vi "search hands data.vi"(11 "offset past number":i32) -> (1 "time delay":i32, 3 "hand":T1 {"手臂" scale=0.0..90.0; "转台" scale=0.0..360.0; "拇指" scale=0.0..90.0; "上下移动" scale=0.0..100.0; "食指" scale=0.0..90.0; "中指" scale=0.0..90.0; "无名指" scale=0.0..90.0; "小手指" scale=0.0..90.0; "手腕" scale=0.0..360.0})   [LabVIEW 2016]
uses:
  Controls/robotdata.ctl
  Data Base/StateMachineStates.ctl
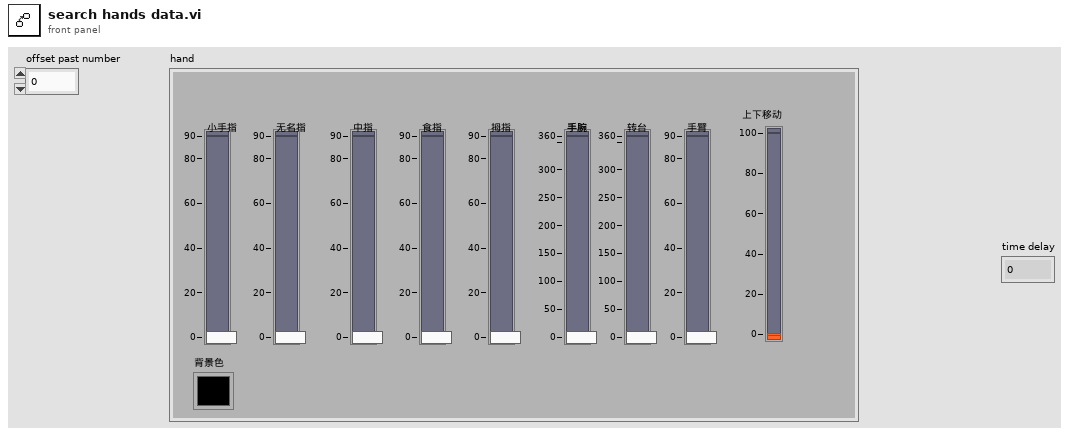
[diagram p1: front panel]
types:
  T1 = typedef "robotdata.ctl" = cluster{"手腕":sgl, "小手指":sgl, "无名指":sgl, "中指":sgl, "食指":sgl, "上下移动":dbl, "背景色":u32, "拇指":sgl, "转台":sgl, "手臂":sgl}
  T2 = typedef "StateMachineStates.ctl" = enum16{"Connection DB", "Creat DB", "Delete Table", "Insert DB", "Inquire Table", "Inquire All DB", "Delete All Data", "Delete Data", "Sort Data", "Inquire Last Data", ""}
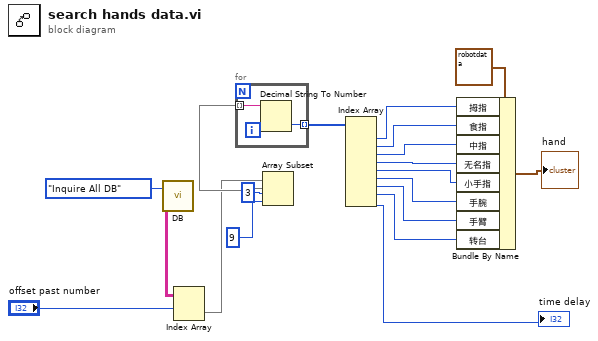
[diagram p0: block diagram]
diagram:
  n1 = call "DB.vi"("Beginning State"=StateMachineStates."Inquire All DB") -> ("Item Data"=w3:string[][])  [unwired: 12 in, 6 out]
  n2 = Index Array(array=w3, index (row)="offset past number") -> (element=w5:string[])  [unwired: 1 in]
  n3 = Array Subset(array=w5, index=3 ("索引"), length=9 ("长度")) -> (w8:string[])
  n4 = for {
    tunnel: w8 -> [w21] mode=indexing
    tunnel: [w20] -> w9 mode=indexing
    n5 = Decimal String To Number(string=w21) -> (number=w20:i32)  [unwired: 2 in, 1 out]
  }
  n6 = Index Array(array=w9) -> (element #1=w11:i32, element #2=w12:i32, element #3=w13:i32, element #4=w14:i32, element #5=w15:i32, element #6=w16:i32, element #7=w17:i32, element #8=w18:i32, element #9=→"time delay":i32)  [unwired: 9 in]
  n7 = Bundle By Name(cluster=T1 {"手腕"=52.38806, "小手指"=0.0, "无名指"=0.0, "中指"=0.0, "食指"=0.0, "上下移动"=-1.8918918918918917, "背景色"=15204350, "拇指"=0.0, "转台"=52.38806, "手臂"=52.38806} ("hand"), "拇指"=w11, "食指"=w12, "中指"=w13, "无名指"=w14, "小手指"=w15, "手腕"=w16, "手臂"=w17, "转台"=w18) -> (→"hand":T1)
